vi "test_mpsse_spi.vi"() -> ()   [LabVIEW 2016]
uses:
  libMPSSE-SPI.lvlib
panel:
  in  "SPI buffer":string="A"
  in  "stop":bool
  in  "loop delay (ms)":u32=10
  out "sizeTransfered":u32
  in  "value":u8 format="%02x"
  in  "dir":u8=64 format="%02x"
  out "GPIO value out":string
  in  "config":T1={"ClockRate"=5000, "LatencyTimer"=255, "configOptions 0-7"=0, "configOptions 8-15"=0, "configOptions 16-23"=0, "configOptions 24-31"=0, "Pin"=0, "reserved"=0}
  out "outBuffer":string
  out "handle out":u32
  in  "index":u32
  out "ftHandle":u32
  out "LocId":u32
  out "Flags":u32
  out "Type":u32
  out "ID":u32
  out "Description":string
  out "Serial number":string
  out "numChannels out":u32
  out "error out":errorcluster
  # "configOptions\nThis member provides a way to enable/disable features\n\tspecific to the protocol that are implemented in the chip\n\tBIT1-0=CPOL-CPHA:\t00 - MODE0 - data captured on rising edge, propagated on falling\n \t\t\t\t\t\t01 - MODE1 - data captured on falling edge, propagated on rising\n \t\t\t\t\t\t10 - MODE2 - data captured on falling edge, propagated on rising\n \t\t\t\t\t\t11 - MODE3 - data captured on rising edge, propagated on falling\n\tBIT4-BIT2: 000 - A/B/C/D_DBUS3=ChipSelect\n\t\t\t : 001 - A/B/C/D_DBUS4=ChipSelect\n \t\t\t : 010 - A/B/C/D_DBUS5=ChipSelect\n \t\t\t : 011 - A/B/C/D_DBUS6=ChipSelect\n \t\t\t : 100 - A/B/C/D_DBUS7=ChipSelect\n \tBIT5: ChipSelect is active high if this bit is 0\n\tBIT6 -BIT31\t\t: Reserved"
  # "0x40 LED"
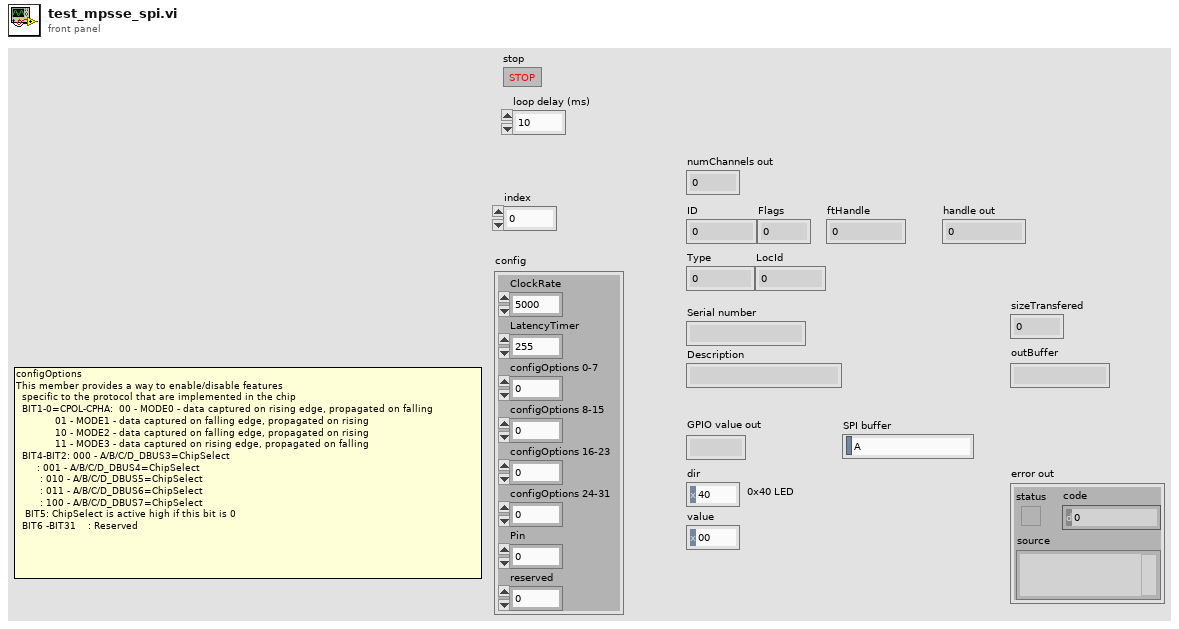
[diagram p1: front panel]
types:
  T1 = cluster{"ClockRate":u32, "LatencyTimer":u8, "configOptions 0-7":i8, "configOptions 8-15":i8, "configOptions 16-23":i8, "configOptions 24-31":u32, "Pin":u32, "reserved":u16}
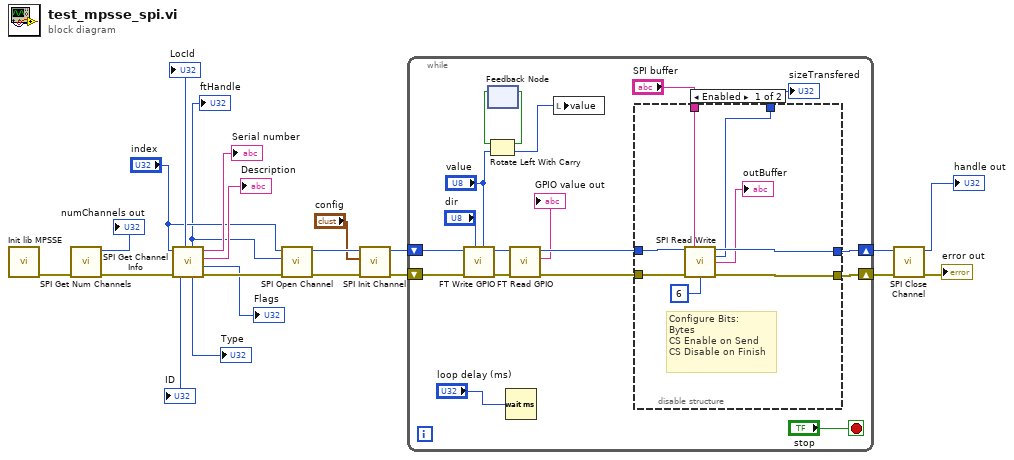
[diagram p0: block diagram]
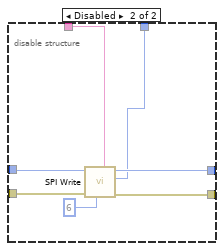
[diagram p2: hidden frame]
diagram:
  n1 = call "Init lib MPSSE.vi"() -> ("error out"=w21:errorcluster)  [unwired: 11 in]
  n2 = call "SPI Get Num Channels.vi"("error in (no error)"=w21) -> ("error out"=w20:errorcluster, "numChannels"=→"numChannels out":u32)  [unwired: 9 in]
  n3 = call "SPI Get Channel Info.vi"("error in (no error)"=w20, "index"="index") -> ("error out"=w16:errorcluster, "Flags"=→"Flags":u32, "Description"=→"Description":string, "Serial number"=→"Serial number":string, "Type"=→"Type":u32, "ftHandle"=w9:u32, "ID"=→"ID":u32, "LocId"=→"LocId":u32)  [unwired: 2 in]
  "ftHandle" <- w9
  n4 = call "SPI Open Channel.vi"("error in (no error)"=w16, "handle"=w9, "index"="index") -> ("error out"=w7:errorcluster, "handle out"=w6:u32)  [unwired: 7 in]
  n5 = call "SPI Init Channel.vi"("error in (no error)"=w7, "config"="config", "handle"=w6) -> ("error out"=w1:errorcluster, "handle out"=w2:u32)  [unwired: 7 in]
  n6 = while {
    shift-right: [w38] -> w3
    shift-left: w2 -> [w36]
    shift-right: [w39] -> w4
    shift-left: w1 -> [w35]
    stop <- "stop" stop-if-true
    n7 = call "FT Write GPIO.vi"("value"="value", "dir"="dir", "error in (no error)"=w35, "handle"=w36) -> ("error out"=w32:errorcluster, "handle out"=w31:u32)  [unwired: 6 in]
    n8 = feedback #1() -> (w26:bool)  [unwired: 1 in]
    n9 = Rotate Left With Carry(2:"value", 3:w26) -> (0:w24:u8, 1:w27:bool)
    n10 = feedback-in #1(w27) -> ()
    n11 = Wait (ms)(milliseconds to wait="loop delay (ms)") -> ()  [unwired: 1 out]
    n12 = call "FT Read GPIO.vi"("error in (no error)"=w32, "handle"=w31) -> ("error out"=w33:errorcluster, "value out"=→"GPIO value out":string, "handle out"=w34:u32)  [unwired: 7 in]
    n13 = local write "value"(w24) -> ()
    n14 = disable-structure shown="Enabled" {
      disable-tunnel: w34 -> [w47 w54]
      disable-tunnel: w33 -> [w46 w53]
      disable-tunnel: [w45 w52] -> w39
      disable-tunnel: [w43 w51] -> w38
      disable-tunnel: "SPI buffer" -> [w41 w49]
      disable-tunnel: [w40 w48] -> w22
      frame Enabled {
        # "Configure Bits:\nBytes\nCS Enable on Send\nCS Disable on Finish"
        n15 = call "SPI Read Write.vi"("handle"=w47, "outBuffer"=w41, "error in (no error)"=w46, "transferOptions"=u32 6) -> ("handle out"=w43:u32, "sizeTransferred"=w40:u32, "inBuffer"=→"outBuffer":string, "error out"=w45:errorcluster)  [unwired: 8 in]
      }
      frame Disabled {
        n16 = call "SPI Write.vi"("buffer"=w49, "options"=u32 6, "error in (no error)"=w53, "handle"=w54) -> ("error out"=w52:errorcluster, "sizeTransfered"=w48:u32, "handle out"=w51:u32)  [unwired: 5 in]
      }
    }
    "sizeTransfered" <- w22
  }
  n17 = call "SPI Close Channel.vi"("error in (no error)"=w4, "handle"=w3) -> ("error out"=→"error out":errorcluster, "handle out"=→"handle out":u32)  [unwired: 7 in, 1 out]
